vi "Demo.vi"() -> ()   [LabVIEW 2010]
panel:
  in  "MVOCX":refnum<k7>(container)
  out "采集BMP图像":picture
  in  "?":bool
  out "采集JPG图像":picture
  in  "Stop":bool
  in  "?":bool
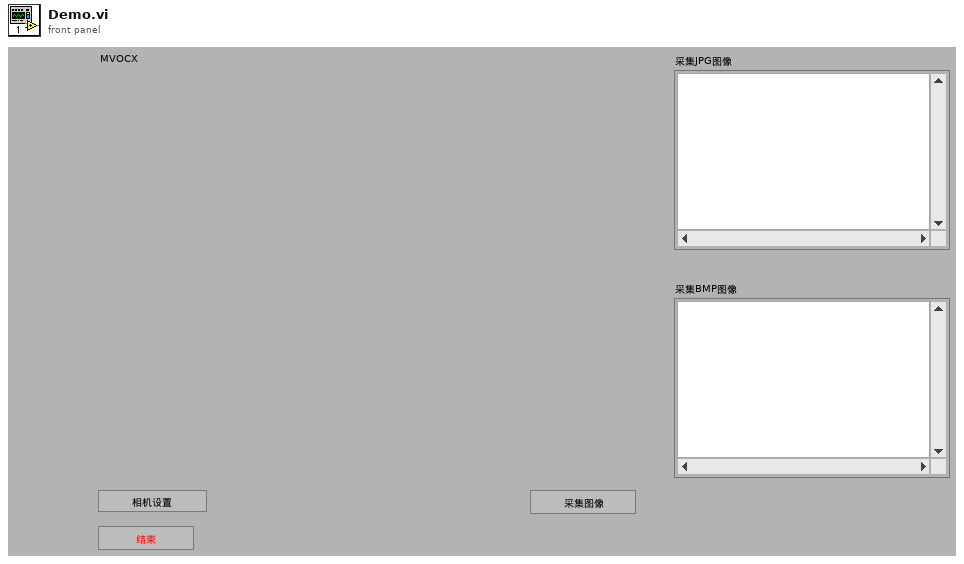
[diagram p1: front panel]
types:
  T1 = typedef "imagedata.ctl" = cluster{"image type":i32, "image depth":i32, "image":u8[], "mask":u8[], "colors":u32[], "Rectangle":cluster{"left":i16, "top":i16, "right":i16, "bottom":i16}}
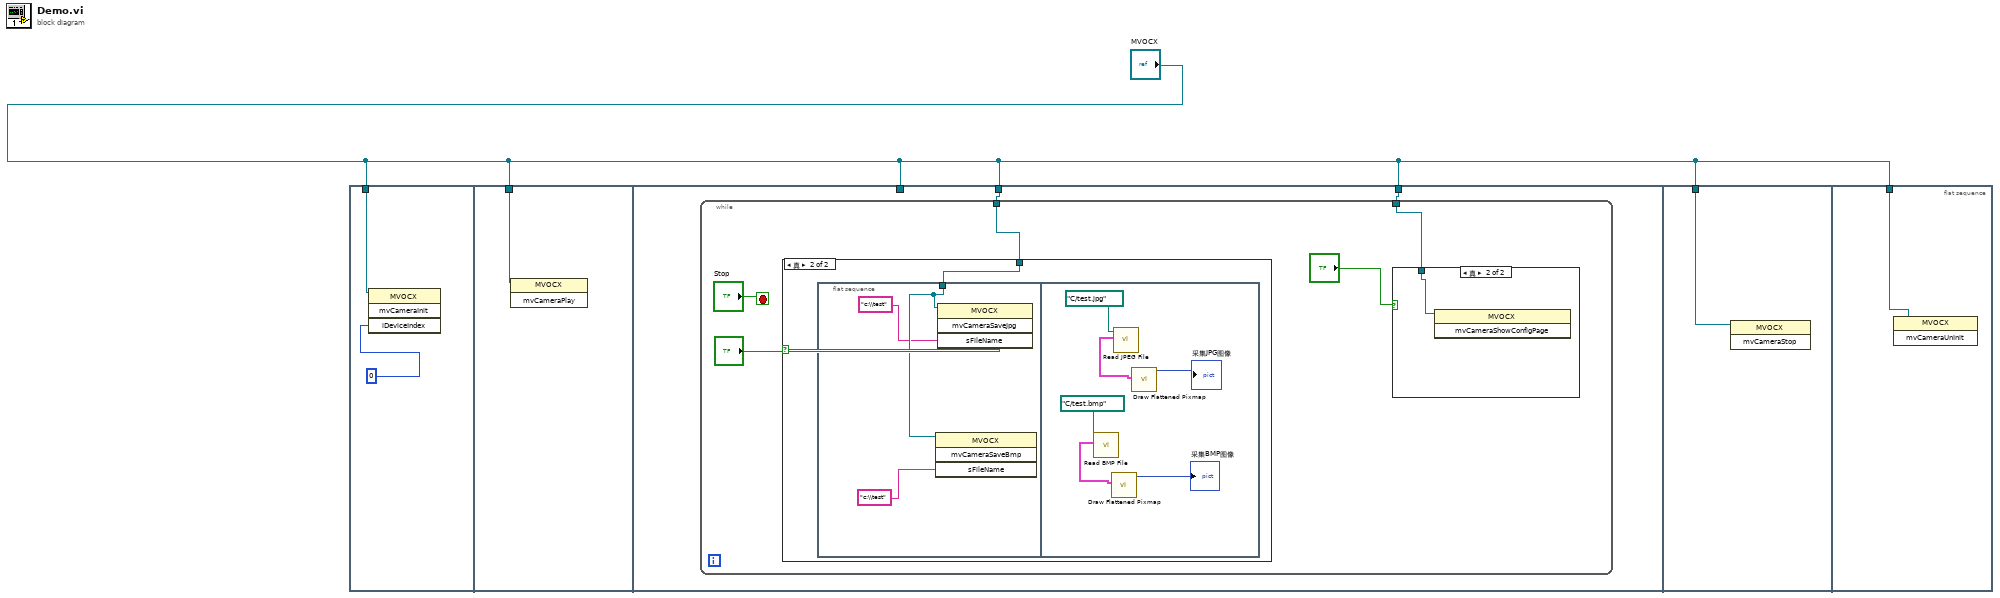
[diagram p0: block diagram]
diagram:
  n1 = flat-sequence {
    tunnel: "MVOCX" -> [w3]
    tunnel: "MVOCX" -> [w4]
    tunnel: "MVOCX" -> [_]
    tunnel: "MVOCX" -> [w6]
    tunnel: "MVOCX" -> [w5]
    tunnel: "MVOCX" -> [w23]
    tunnel: "MVOCX" -> [w24]
    frame #0 {
      n2 = invoke class="MVOCX" method="mvCameraInit"(reference=w3, "iDeviceIndex"=0) -> ()  [unwired: 2 in, 4 out]
    }
    frame #1 {
      n3 = invoke class="MVOCX" method="mvCameraPlay"(reference=w4) -> ()  [unwired: 2 in, 3 out]
    }
    frame #2 {
      n4 = while {
        tunnel: w6 -> [w7]
        tunnel: w5 -> [w8]
        stop <- "Stop" stop-if-true
        n5 = case shown="真" "?" {
          tunnel: w8 -> [_ w13]
          frame False {
          }
          frame True {
            n6 = flat-sequence {
              tunnel: w13 -> [w16]
              frame #0 {
                n7 = invoke class="MVOCX" method="mvCameraSaveBmp"(reference=w16, "sFileName"="c:\\test") -> ()  [unwired: 2 in, 4 out]
                n8 = invoke class="MVOCX" method="mvCameraSaveJpg"(reference=w16, "sFileName"="c:\\test") -> ()  [unwired: 2 in, 4 out]
              }
              frame #1 {
                n9 = call <vilib>:"Read BMP File.vi"("path to BMP file"=path "C:/test.bmp") -> ("image data"=w18:T1)  [unwired: 8 in, 2 out]
                n10 = call <vilib>:"Draw Flattened Pixmap.vi"("image data"=w18) -> ("new picture"=→"采集BMP图像":picture)  [unwired: 8 in]
                n11 = call <vilib>:"Read JPEG File.vi"("path to JPEG file"=path "C:/test.jpg" ("path to BMP file")) -> ("image data"=w21:T1)  [unwired: 8 in, 2 out]
                n12 = call <vilib>:"Draw Flattened Pixmap.vi"("image data"=w21) -> ("new picture"=→"采集JPG图像":picture)  [unwired: 8 in]
              }
            }
          }
        }
        n13 = case shown="真" "?" {
          tunnel: w7 -> [_ w12]
          frame False {
          }
          frame True {
            n14 = invoke class="MVOCX" method="mvCameraShowConfigPage"(reference=w12) -> ()  [unwired: 2 in, 3 out]
          }
        }
      }
    }
    frame #3 {
      n15 = invoke class="MVOCX" method="mvCameraStop"(reference=w23) -> ()  [unwired: 2 in, 3 out]
    }
    frame #4 {
      n16 = invoke class="MVOCX" method="mvCameraUnInit"(reference=w24) -> ()  [unwired: 2 in, 3 out]
    }
  }
